vi "midi out open.vi"(7 "UDeviceID":i32) -> (0 "Win32 error code":i32, 3 "Hmidiout handle":i32)   [LabVIEW 2016]
doc: "Opens a reference to a MIDI output device."
uses:
  winmm.dll
panel:
  # "Select Help»Show Context Help and move the cursor over the VI icon to display help for this VI."
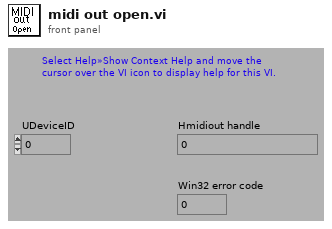
[diagram p1: front panel]
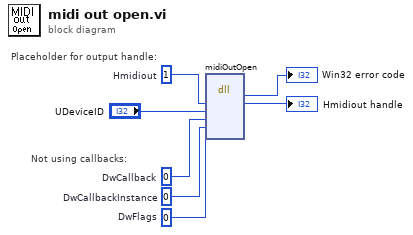
[diagram p0: block diagram]
diagram:
  w1 = 0  # DwFlags
  w2 = 0  # DwCallbackInstance
  w3 = 0  # DwCallback
  w5 = 1  # Hmidiout
  # "Placeholder for output handle:"
  # "Not using callbacks:"
  n1 = dll-call lib="winmm.dll" fn="midiOutOpen"("hmidiout"=w5, "uDeviceID"="UDeviceID", "dwCallback"=w3, "dwCallbackInstance"=w2, "dwFlags"=w1) -> (→"Win32 error code":i32, "hmidiout"=→"Hmidiout handle":i32)  [unwired: 7 in, 2 out]
